vi "HorzLines.vi"(6 "Spacing":dbl, 8 "yMax":dbl, 9 "yMin":dbl, 10 "xMax":dbl, 11 "xMin":dbl) -> (2 "Poly2D":T1, 3 "Pnts":sgl[][](array[numeric]))   [LabVIEW 2014]
uses:
  TypeDefs/Poly2DwSlope.ctl
  TypeDefs/Point2DwSlope.ctl
panel:
  out "XY Graph":T3(graph)
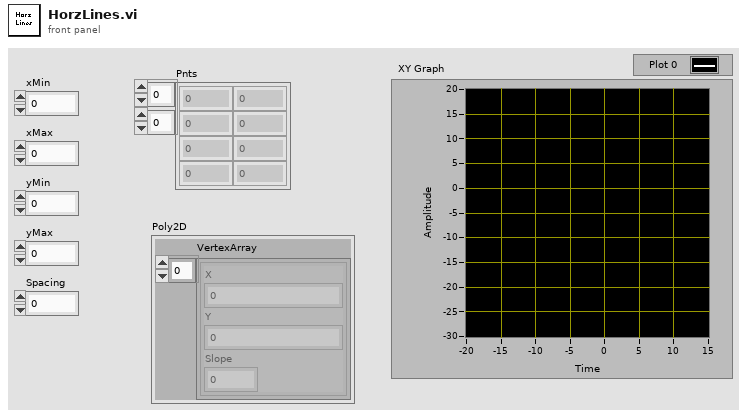
[diagram p1: front panel]
types:
  T1 = typedef "Poly2DwSlope.ctl" = cluster{"VertexArray":T2[]}
  T2 = typedef "Point2DwSlope.ctl" = cluster{"X":sgl, "Y":sgl, "Slope":dbl}
  T3 = cluster{"VertexArray":cluster{"X":sgl, "Y":sgl, "Slope":dbl}[]}[]
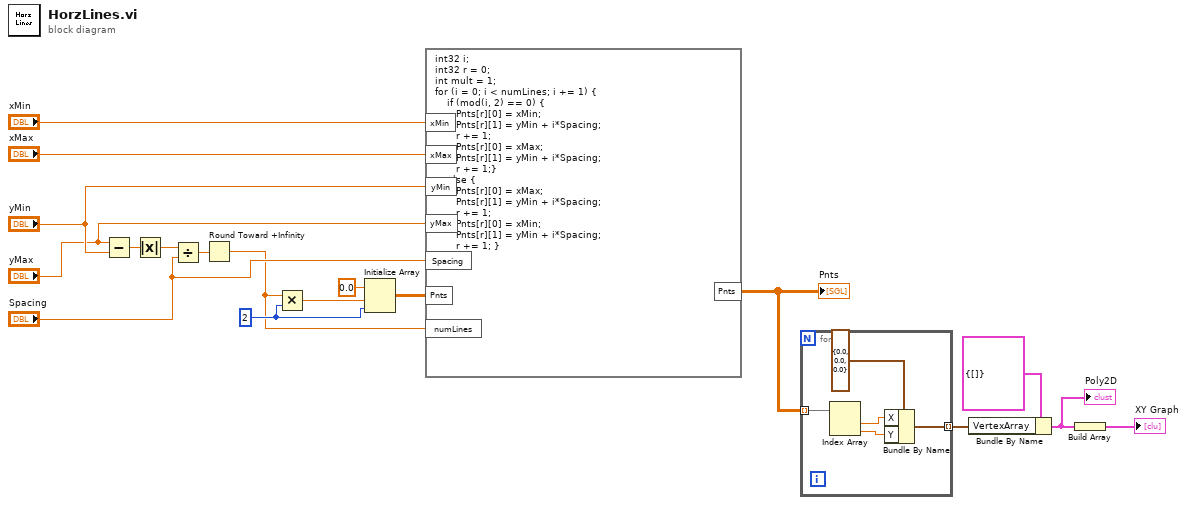
[diagram p0: block diagram]
diagram:
  w13 = 2 ("dimension size")
  n1 = Subtract(x="yMax", y="yMin") -> (x-y=w16:dbl)
  n2 = Absolute Value(x=w16) -> (abs(x)=w15:dbl)
  n3 = Divide(x=w15, y="Spacing") -> (x/y=w14:dbl)
  n4 = Round Toward +Infinity(x=w14) -> (ceil(x): smallest int >= x=w6:dbl)
  n5 = Multiply(x=w6, y=w13) -> (x*y=w12:dbl)
  n6 = Initialize Array(sgl 0.0 ("element"), w12, w13) -> (w17:sgl[][])
  n7 = formula code="int32 i;\nint32 r = 0;\nint mult = 1;\nfor (i = 0; i < numLines; i += 1) {\n    if (mod(i, 2) == 0) {\n       Pnts[r][0] = xMin;\n       Pnts[r][1] = yMin + i*Spacing;\n       r += 1;\n       Pnts[r][0] = xMax;\n       Pnts[r][1] = yMin + i*Spacing;\n       r += 1;}\n    else {\n       Pnts[r][0] = xMax;\n       Pnts[r][1] = yMin + i*Spacing;\n       r += 1;\n       Pnts[r][0] = xMin;\n       Pnts[r][1] = yMin + i*Spacing;\n       r += 1; }\n    }"("xMin"="xMin", "xMax"="xMax", "yMin"="yMin", "yMax"="yMax", "Spacing"="Spacing", "Pnts"=w17, "numLines"=w6) -> ("Pnts"=w5:sgl[][])
  "Pnts" <- w5
  n8 = for {
    tunnel: w5 -> [w22] mode=indexing
    tunnel: [w19] -> w3 mode=indexing
    n9 = Index Array(array=w22) -> (element #1=w21:sgl, element #2=w20:sgl)  [unwired: 2 in]
    n10 = Bundle By Name(cluster=T2 {"X"=0.0, "Y"=0.0, "Slope"=0.0} ("Point2D"), "X"=w21, "Y"=w20) -> (w19:T2)
  }
  n11 = Bundle By Name(cluster=T1 {"VertexArray"=[]} ("Poly2D"), "VertexArray"=w3) -> (w1:T1)
  "Poly2D" <- w1
  n12 = Build Array(w1) -> (→"XY Graph":T1[])
